vi "OrdenarPosDefesa.vi"(8 "geometry":T1, 11 "Posições da defesa":dbl[][](array[numeric]) format="%#_13g") -> (1 "Pos ordenada 3":dbl[](array[numeric]) format="%#_13g", 2 "Pos ordenada 2":dbl[](array[numeric]) format="%#_13g", 3 "Pos ordenada 1":dbl[](array[numeric]) format="%#_13g")   [LabVIEW 2017]
uses:
  Core/Field Size.ctl
  148dee89-422f-4aae-9114-a40a4011e594.vi
  <vilib>/Array/Sort 2D Array - Pop Stack.vi
  <vilib>/Array/Sort 2D Array - Push Stack.vi
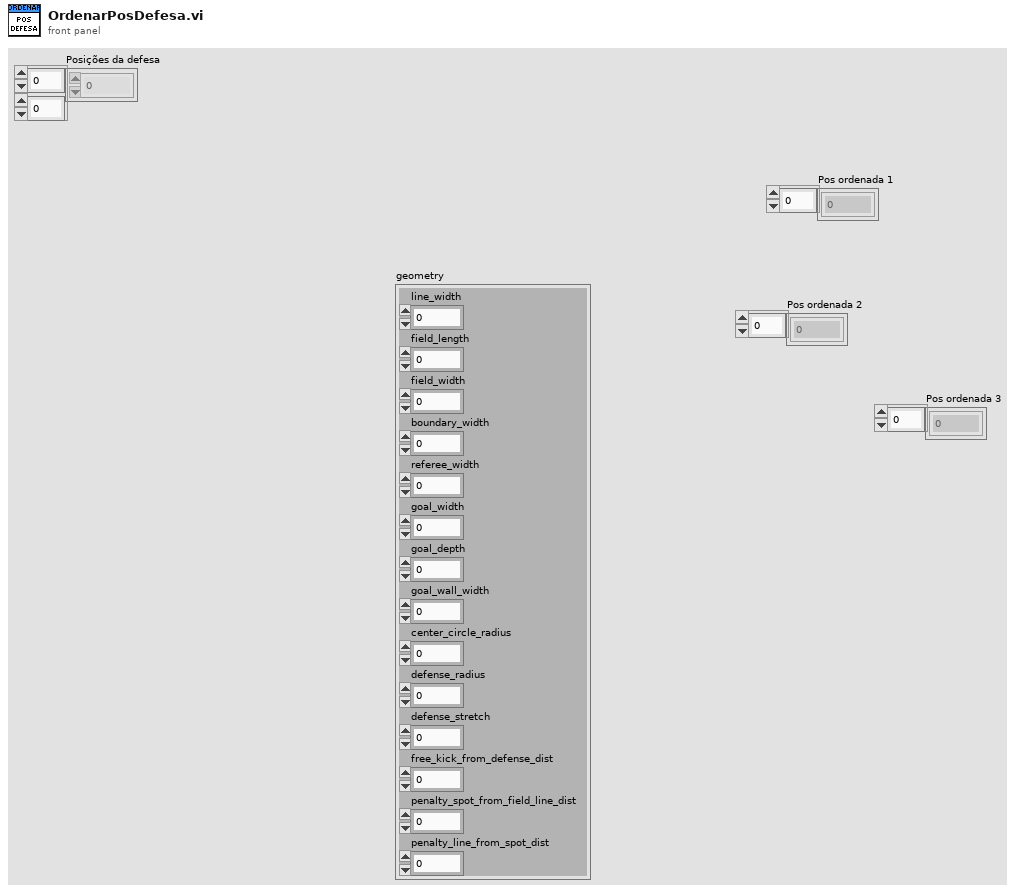
[diagram p1: front panel]
types:
  T1 = typedef "Field Size.ctl" = cluster{"line_width":u32, "field_length":u32, "field_width":u32, "boundary_width":u32, "referee_width":u32, "goal_width":u32, "goal_depth":u32, "goal_wall_width":u32, "center_circle_radius":u32, "defense_radius":u32, "defense_stretch":u32, "free_kick_from_defense_dist":u32, "penalty_spot_from_field_line_dist":u32, "penalty_line_from_spot_dist":u32}
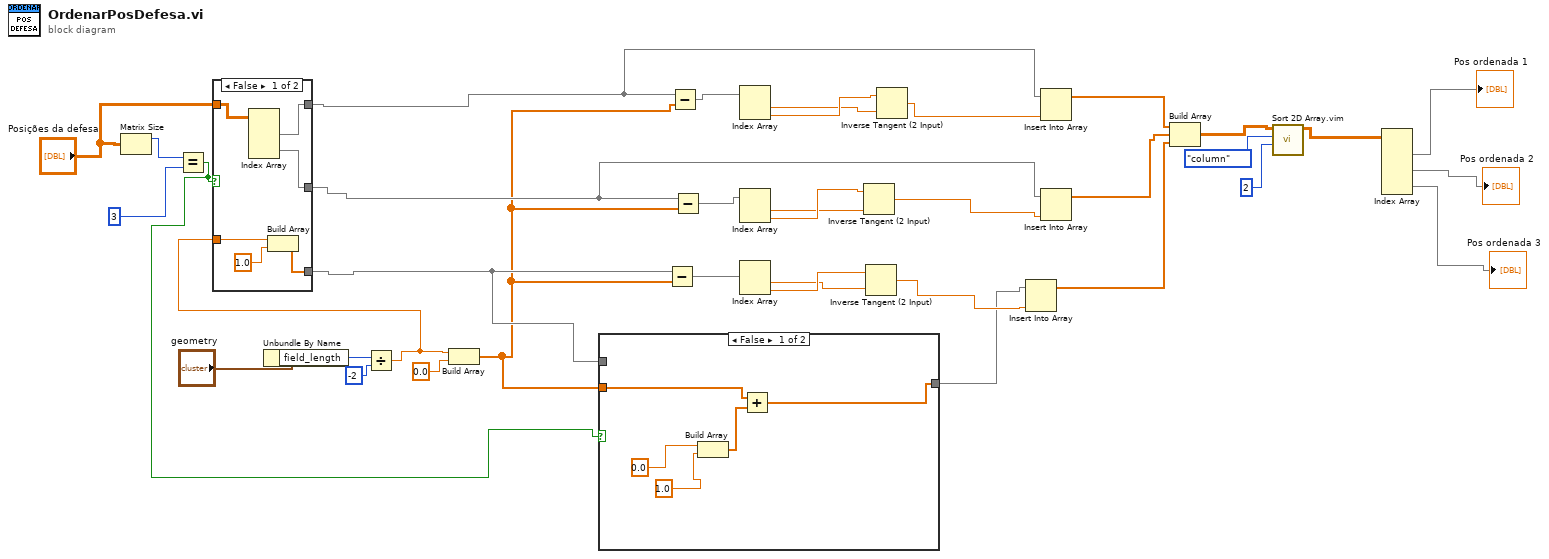
[diagram p0: block diagram]
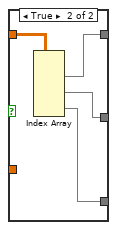
[diagram p3: hidden frame]
diagram:
  n1 = Matrix Size(0:"Posições da defesa") -> (1:w1:i32)  [unwired: 1 out]
  n2 = Equal?(x=w1, y=3) -> (x = y?=w6:bool)
  n3 = Unbundle By Name("geometry") -> ("field_length"=w35:u32)
  n4 = Divide(x=w35, y=-2) -> (x/y=w7:dbl)
  n5 = case shown="False" w6 {
    tunnel: "Posições da defesa" -> [w42 w46]
    tunnel: [w41 w45] -> w9
    tunnel: [w40 w44] -> w8
    tunnel: [w38 w43] -> w4
    tunnel: w7 -> [w37 _]
    frame False {
      n6 = Index Array(array=w42) -> (element #1=w41:dbl[], element #2=w40:dbl[])  [unwired: 4 in]
      n7 = Build Array(w37, 1.0) -> (w38:dbl[])
    }
    frame True {
      n8 = Index Array(array=w46) -> (element #1=w45:dbl[], element #2=w44:dbl[], element #3=w43:dbl[])  [unwired: 6 in]
    }
  }
  n9 = Build Array(w7, 0.0 ("element")) -> (w3:dbl[])
  n10 = case shown="False" w6 {
    tunnel: [w47 w52] -> w5
    tunnel: w4 -> [_ w52]
    tunnel: w3 -> [w51 _]
    frame False {
      n11 = Build Array(0.0, 1.0) -> (w48:dbl[])
      n12 = Add(x=w51, y=w48) -> (x+y=w47:dbl[])
    }
    frame True {
    }
  }
  n13 = Subtract(x=w4, y=w3) -> (x-y=w30:dbl[])
  n14 = Subtract(x=w9, y=w3) -> (x-y=w32:dbl[])
  n15 = Subtract(x=w8, y=w3) -> (x-y=w31:dbl[])
  n16 = Index Array(array=w32) -> (element #1=w28:dbl, element #2=w29:dbl)  [unwired: 2 in]
  n17 = Index Array(array=w31) -> (element #1=w26:dbl, element #2=w27:dbl)  [unwired: 2 in]
  n18 = Index Array(array=w30) -> (element #1=w24:dbl, element #2=w25:dbl)  [unwired: 2 in]
  n19 = Inverse Tangent (2 Input)(1:w26, 2:w27) -> (0:w22:dbl)
  n20 = Inverse Tangent (2 Input)(1:w24, 2:w25) -> (0:w21:dbl)
  n21 = Inverse Tangent (2 Input)(1:w28, 2:w29) -> (0:w23:dbl)
  n22 = Insert Into Array(array=w5, new element=w21) -> (w18:dbl[])  [unwired: 1 in]
  n23 = Insert Into Array(array=w9, new element=w23) -> (w20:dbl[])  [unwired: 1 in]
  n24 = Insert Into Array(array=w8, new element=w22) -> (w19:dbl[])  [unwired: 1 in]
  n25 = Build Array(w20, w19, w18) -> (w17:dbl[][])
  n26 = call "Sort 2D Array.vim"("index"=2, "dimension to index (column)"=enum16{"column", "row"}."column", "2D array"=w17) -> ("sorted 2D array"=w14:dbl[][])  [unwired: 7 in, 1 out]
  n27 = Index Array(array=w14) -> (element #1=→"Pos ordenada 1":dbl[], element #2=→"Pos ordenada 2":dbl[], element #3=→"Pos ordenada 3":dbl[])  [unwired: 6 in]
